vi "ROIText.vi"(11 "ROI":T1) -> (0 "draw":string, 1 "with comma":string, 2 "roi = r":string, 3 "r":string)   [LabVIEW 2020]
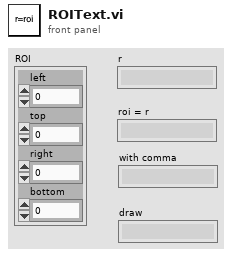
[diagram p1: front panel]
types:
  T1 = cluster{"left":i32, "top":i32, "right":i32, "bottom":i32}
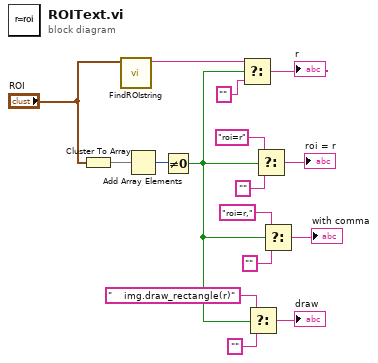
[diagram p0: block diagram]
diagram:
  n1 = Cluster To Array(cluster="ROI") -> (array=w8:i32[])
  n2 = call "FindROIstring.vi"("ROI"="ROI") -> ("String"=w10:string)  [unwired: 9 in, 1 out]
  n3 = Add Array Elements(numeric array=w8) -> (sum=w9:i32)
  n4 = Not Equal To 0?(x=w9) -> (x != 0?=w1:bool)
  n5 = Select(t=w10, s=w1, f="") -> (s? t:f=→"r":string)
  n6 = Select(t="    img.draw_rectangle(r)" ("f"), s=w1, f="") -> (s? t:f=→"draw":string)
  n7 = Select(t="roi=r" ("f"), s=w1, f="") -> (s? t:f=→"roi = r":string)
  n8 = Select(t="roi=r," ("f"), s=w1, f="") -> (s? t:f=→"with comma":string)
